vi "Analyse error.vi"(8 "error in (no error)":errorcluster, 11 "IErrorHandler in":refnum<class "AbortHandler JSON.lvclass">) -> (0 "error out":errorcluster, 3 "IErrorHandler out":refnum<class "AbortHandler JSON.lvclass">)   [LabVIEW 2020, in "wamplv.lvlib" / "AbortHandler JSON.lvclass"]
uses:
  AbortHandler JSON.lvclass
  AbortHandler JSON.lvclass/AbortHandler JSON.ctl
  Utils/Utils.lvclass
  <vilib>/Utility/error.llb/Error Cluster From Error Code.vi
  <vilib>/ErrorRing/Error Ring.xnode
  wamplv.lvlib
  SerialisedMessages/JSONMessage/WampMessage JSON.lvclass
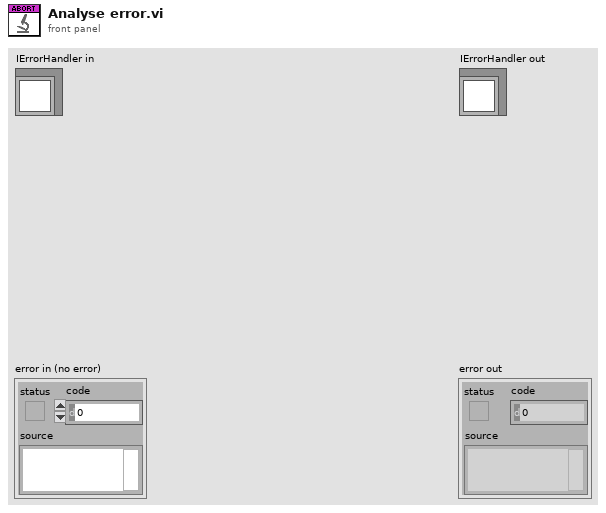
[diagram p1: front panel]
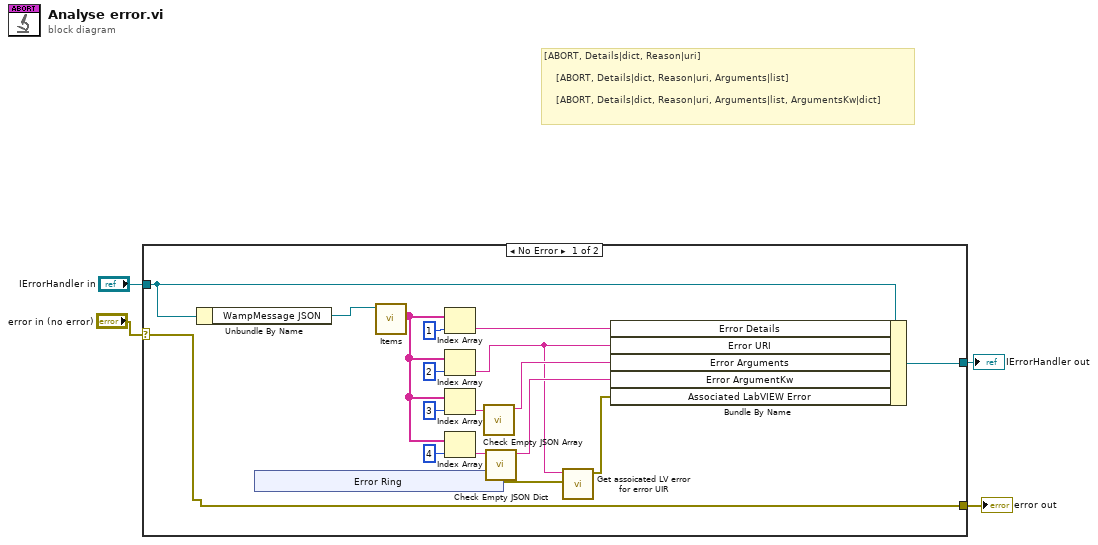
[diagram p0: block diagram]
diagram:
  # "[ABORT, Details|dict, Reason|uri]\n\n    [ABORT, Details|dict, Reason|uri, Arguments|list]\n\n    [ABORT, Details|dict, Reason|uri, Arguments|list, ArgumentsKw|dict]"
  n1 = case shown="No Error" "error in (no error)" {
    selector: "error in (no error)" -> [w5 w26]
    tunnel: "IErrorHandler in" -> [w6 w27]
    tunnel: [w11 w27] -> w2
    tunnel: [w5 w26] -> w1
    frame No Error {
      n2 = Unbundle By Name(w6) -> ("WampMessage JSON"=w7:refnum<class "WampMessage JSON.lvclass">)
      n3 = xnode "Error Ring"() -> ("error out"=w10:errorcluster)
      n4 = call-dynamic "Items.vi"("JSONMessage in"=w7) -> ("<JSON>Elements"=w16:string[])  [unwired: 9 in, 1 out]
      n5 = Index Array(array=w16, index=1) -> (element=w20:string)
      n6 = Index Array(array=w16, index=2) -> (element=w9:string)
      n7 = Index Array(array=w16, index=3) -> (element=w15:string)
      n8 = Index Array(array=w16, index=4) -> (element=w13:string)
      n9 = call "Check Empty JSON Array.vi"("JSON in"=w15) -> ("JSON out"=w14:string)  [unwired: 10 in]
      n10 = call "Check Empty JSON Dict.vi"("JSON in"=w13) -> ("JSON out"=w12:string)  [unwired: 10 in]
      n11 = call "Get assoicated LV error for error UIR.vi"("Default error"=w10, "URI"=w9) -> ("Associated error"=w8:errorcluster)  [unwired: 9 in]
      n12 = Bundle By Name(cluster=w6, "Error Details"=w20, "Error URI"=w9, "Error Arguments"=w14, "Error ArgumentKw"=w12, "Associated LabVIEW Error"=w8) -> (w11:refnum<class "AbortHandler JSON.lvclass">)
    }
    frame Error {
    }
  }
  "error out" <- w1
  "IErrorHandler out" <- w2
